vi "Queue Priority TEST.vi"() -> ()   [LabVIEW 2023]
uses:
  Queues.lvlib
  DUTResult.ctl
  Queue Priority.ctl
  DUTinfo.ctl
panel:
  out "secfond element":T1
  out "first element":T1
  out "error out":errorcluster
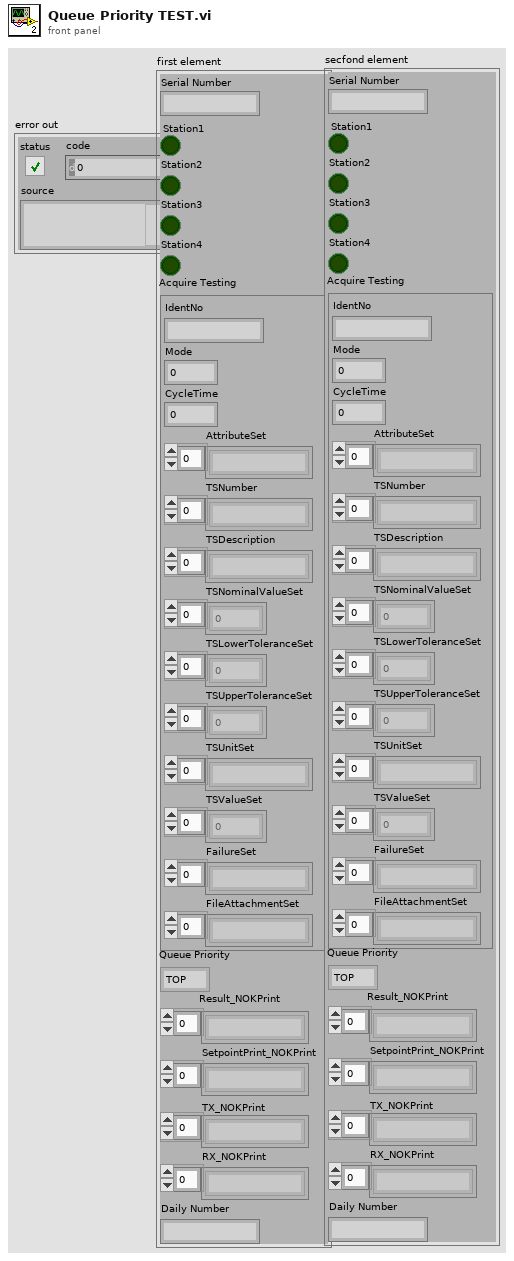
[diagram p1: front panel]
types:
  T1 = typedef "Queues.lvlib/DUTinfo.ctl" = cluster{"Serial Number":string, "Station1":bool, "Station2":bool, "Station3":bool, "Station4":bool, "Acquire Testing":T2, "Queue Priority":T3, "Result_NOKPrint":string[], "SetpointPrint_NOKPrint":string[], "TX_NOKPrint":string[], "RX_NOKPrint":string[], "Daily Number":string}
  T2 = typedef "Queues.lvlib/DUTResult.ctl" = cluster{"IdentNo":string, "Mode":dbl, "CycleTime":dbl, "AttributeSet":string[], "TSNumber":string[], "TSDescription":string[], "TSNominalValueSet":dbl[], "TSLowerToleranceSet":dbl[], "TSUpperToleranceSet":dbl[], "TSUnitSet":string[], "TSValueSet":dbl[], "FailureSet":string[], "FileAttachmentSet":string[]}
  T3 = typedef "Queues.lvlib/Queue Priority.ctl" = enum16{"TOP", "BOTTOM"}
  T4 = typedef "Queues.lvlib/DUTinfo.ctl" = cluster{"Serial Number":string, "Variant":string, "LOADING":bool, "EOLA":bool, "EOLB":bool, "EOLC":bool, "PIN CHECK":bool, "LABELING":bool, "Acquire Testing":T2, "Queue Priority":T3, "Result_NOKPrint":string[], "SetpointPrint_NOKPrint":string[], "TX_NOKPrint":string[], "RX_NOKPrint":string[], "Daily Number":string}
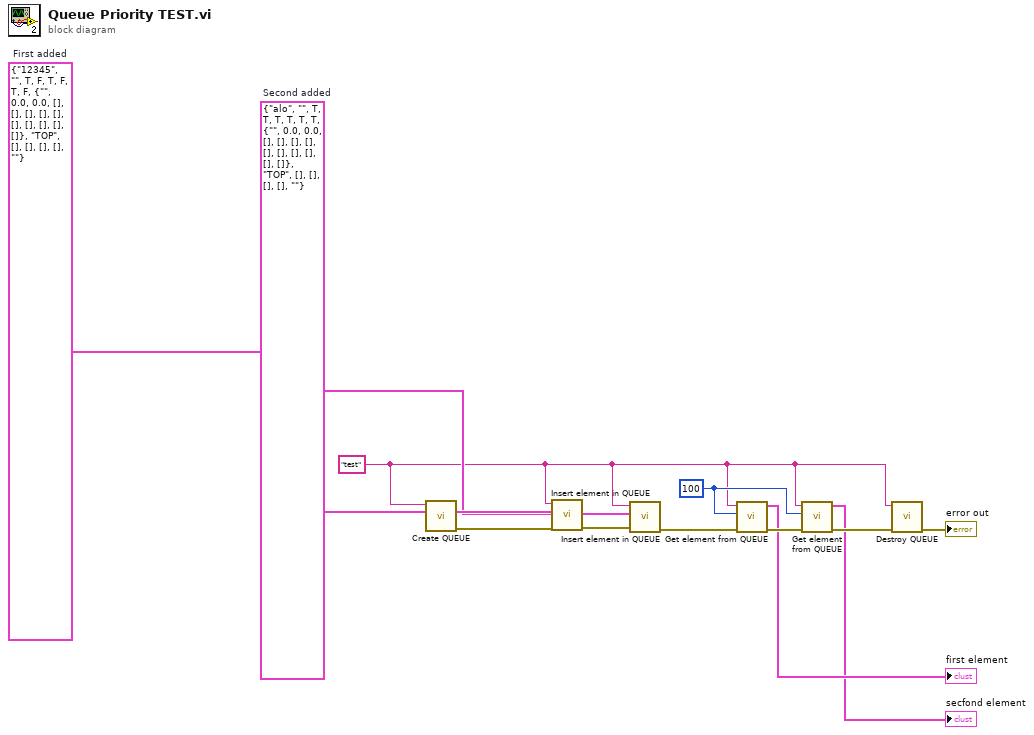
[diagram p0: block diagram]
diagram:
  w5 = 100 ("timeout in ms")
  w9 = T4 {"Serial Number"="alo", "Variant"="", "LOADING"=TRUE, "EOLA"=TRUE, "EOLB"=TRUE, "EOLC"=TRUE, "PIN CHECK"=TRUE, "LABELING"=TRUE, "Acquire Testing"={"IdentNo"="", "Mode"=0.0, "CycleTime"=0.0, "AttributeSet"=[], "TSNumber"=[], "TSDescription"=[], "TSNominalValueSet"=[], "TSLowerToleranceSet"=[], "TSUpperToleranceSet"=[], "TSUnitSet"=[], "TSValueSet"=[], "FailureSet"=[], "FileAttachmentSet"=[]}, "Queue Priority"=enum."TOP", "Result_NOKPrint"=[], "SetpointPrint_NOKPrint"=[], "TX_NOKPrint"=[], "RX_NOKPrint"=[], "Daily Number"=""}  # Second added
  w11 = T4 {"Serial Number"="12345", "Variant"="", "LOADING"=TRUE, "EOLA"=FALSE, "EOLB"=TRUE, "EOLC"=FALSE, "PIN CHECK"=TRUE, "LABELING"=FALSE, "Acquire Testing"={"IdentNo"="", "Mode"=0.0, "CycleTime"=0.0, "AttributeSet"=[], "TSNumber"=[], "TSDescription"=[], "TSNominalValueSet"=[], "TSLowerToleranceSet"=[], "TSUpperToleranceSet"=[], "TSUnitSet"=[], "TSValueSet"=[], "FailureSet"=[], "FileAttachmentSet"=[]}, "Queue Priority"=enum."TOP", "Result_NOKPrint"=[], "SetpointPrint_NOKPrint"=[], "TX_NOKPrint"=[], "RX_NOKPrint"=[], "Daily Number"=""}  # First added
  w1 = "test" ("QueueName")
  n1 = call "Create QUEUE.vi"("QueueName"=w1) -> ("error out"=w12:errorcluster)  [unwired: 8 in, 1 out]
  n2 = call "Insert element in QUEUE.vi"("error in (no error)"=w12, "Element"=w11, "Queue name"=w1) -> ("error out"=w10:errorcluster)  [unwired: 7 in, 1 out]
  n3 = call "Insert element in QUEUE.vi"("error in (no error)"=w10, "Element"=w9, "Queue name"=w1) -> ("error out"=w7:errorcluster)  [unwired: 7 in, 1 out]
  n4 = call "Get element from QUEUE.vi"("error in (no error)"=w7, "timeout in ms"=w5, "Queue Name"=w1) -> ("error out"=w6:errorcluster, "element"=→"first element":T1)  [unwired: 5 in, 1 out]
  n5 = call "Get element from QUEUE.vi"("error in (no error)"=w6, "timeout in ms"=w5, "Queue Name"=w1) -> ("error out"=w4:errorcluster, "element"=→"secfond element":T1)  [unwired: 5 in, 1 out]
  n6 = call "Destroy QUEUE.vi"("error in (no error)"=w4, "Queue name"=w1) -> ("error out"=→"error out":errorcluster)  [unwired: 9 in]
